vi "Akustische Füllstandsanzeige.vi"() -> ()   [LabVIEW 2018]
uses:
  <vilib>/measure/maspectr.llb/FFT Power Spectrum and PSD for 1 Chan.vi
  <vilib>/measure/NI_MAPro.lvlib
panel:
  out "?":dbl
  out "FFT-Leistung":cluster{"f0":dbl, "df":dbl, "magnitude":dbl[]}(graph)
  in  "Auswahl Gefäß":u16(ring)
  out "?":dbl(slide) scale=0.0..200.0
  in  "?":bool
  # "Füllstand in ml"
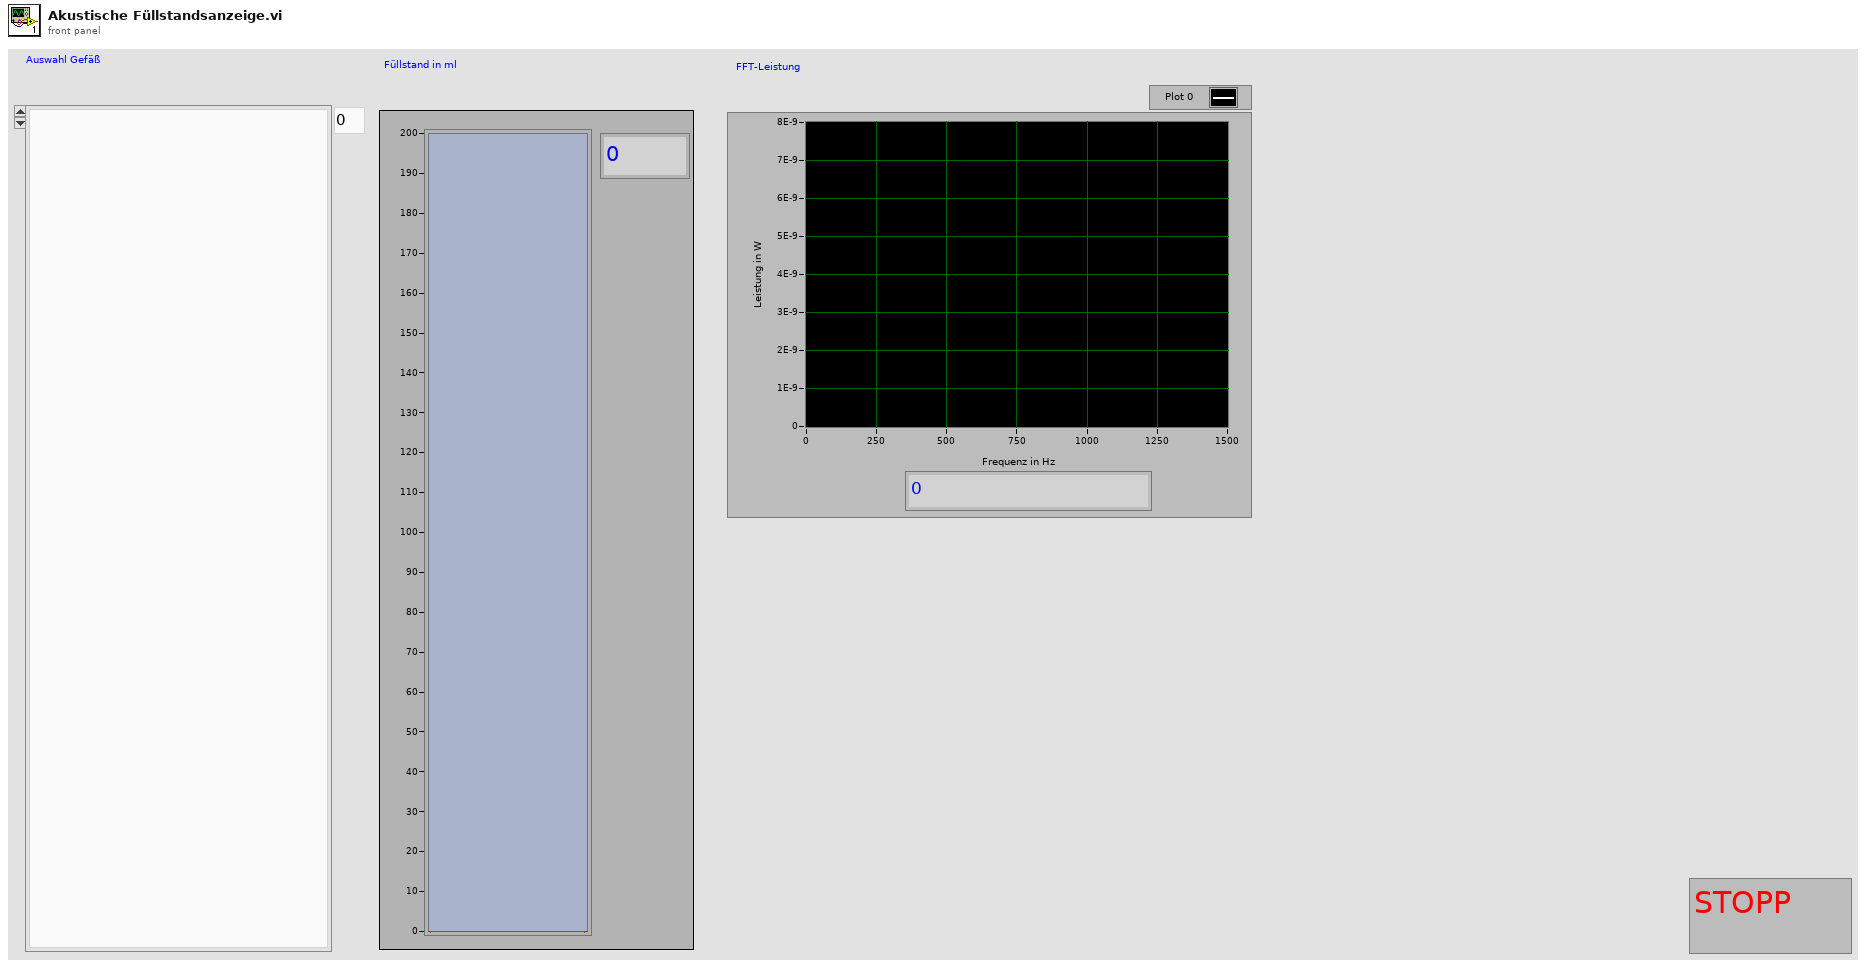
[diagram p1: front panel]
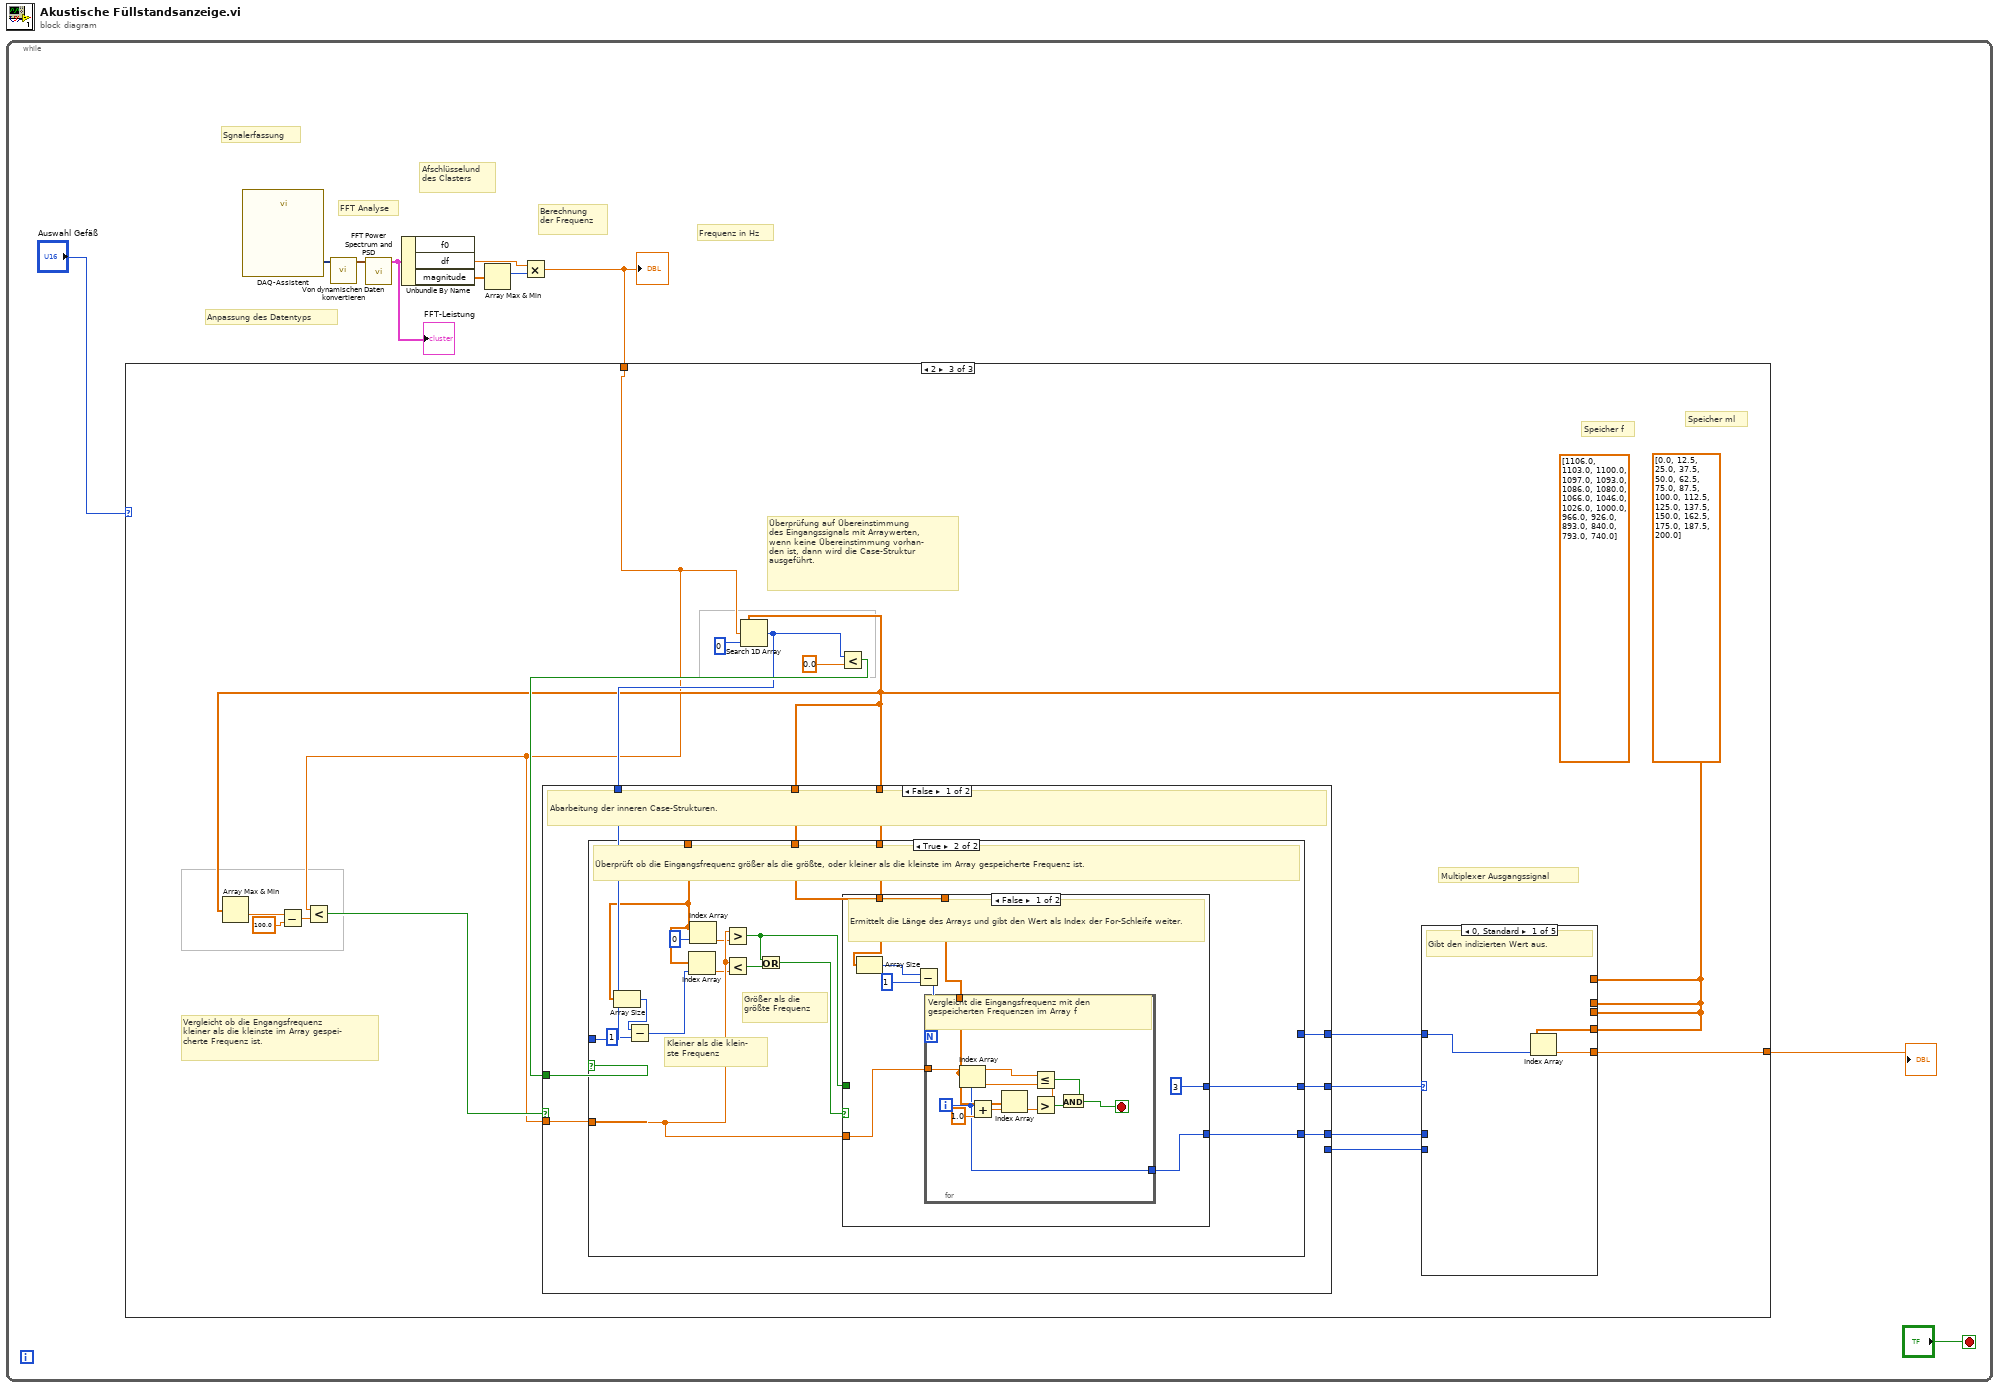
[diagram p0: block diagram]
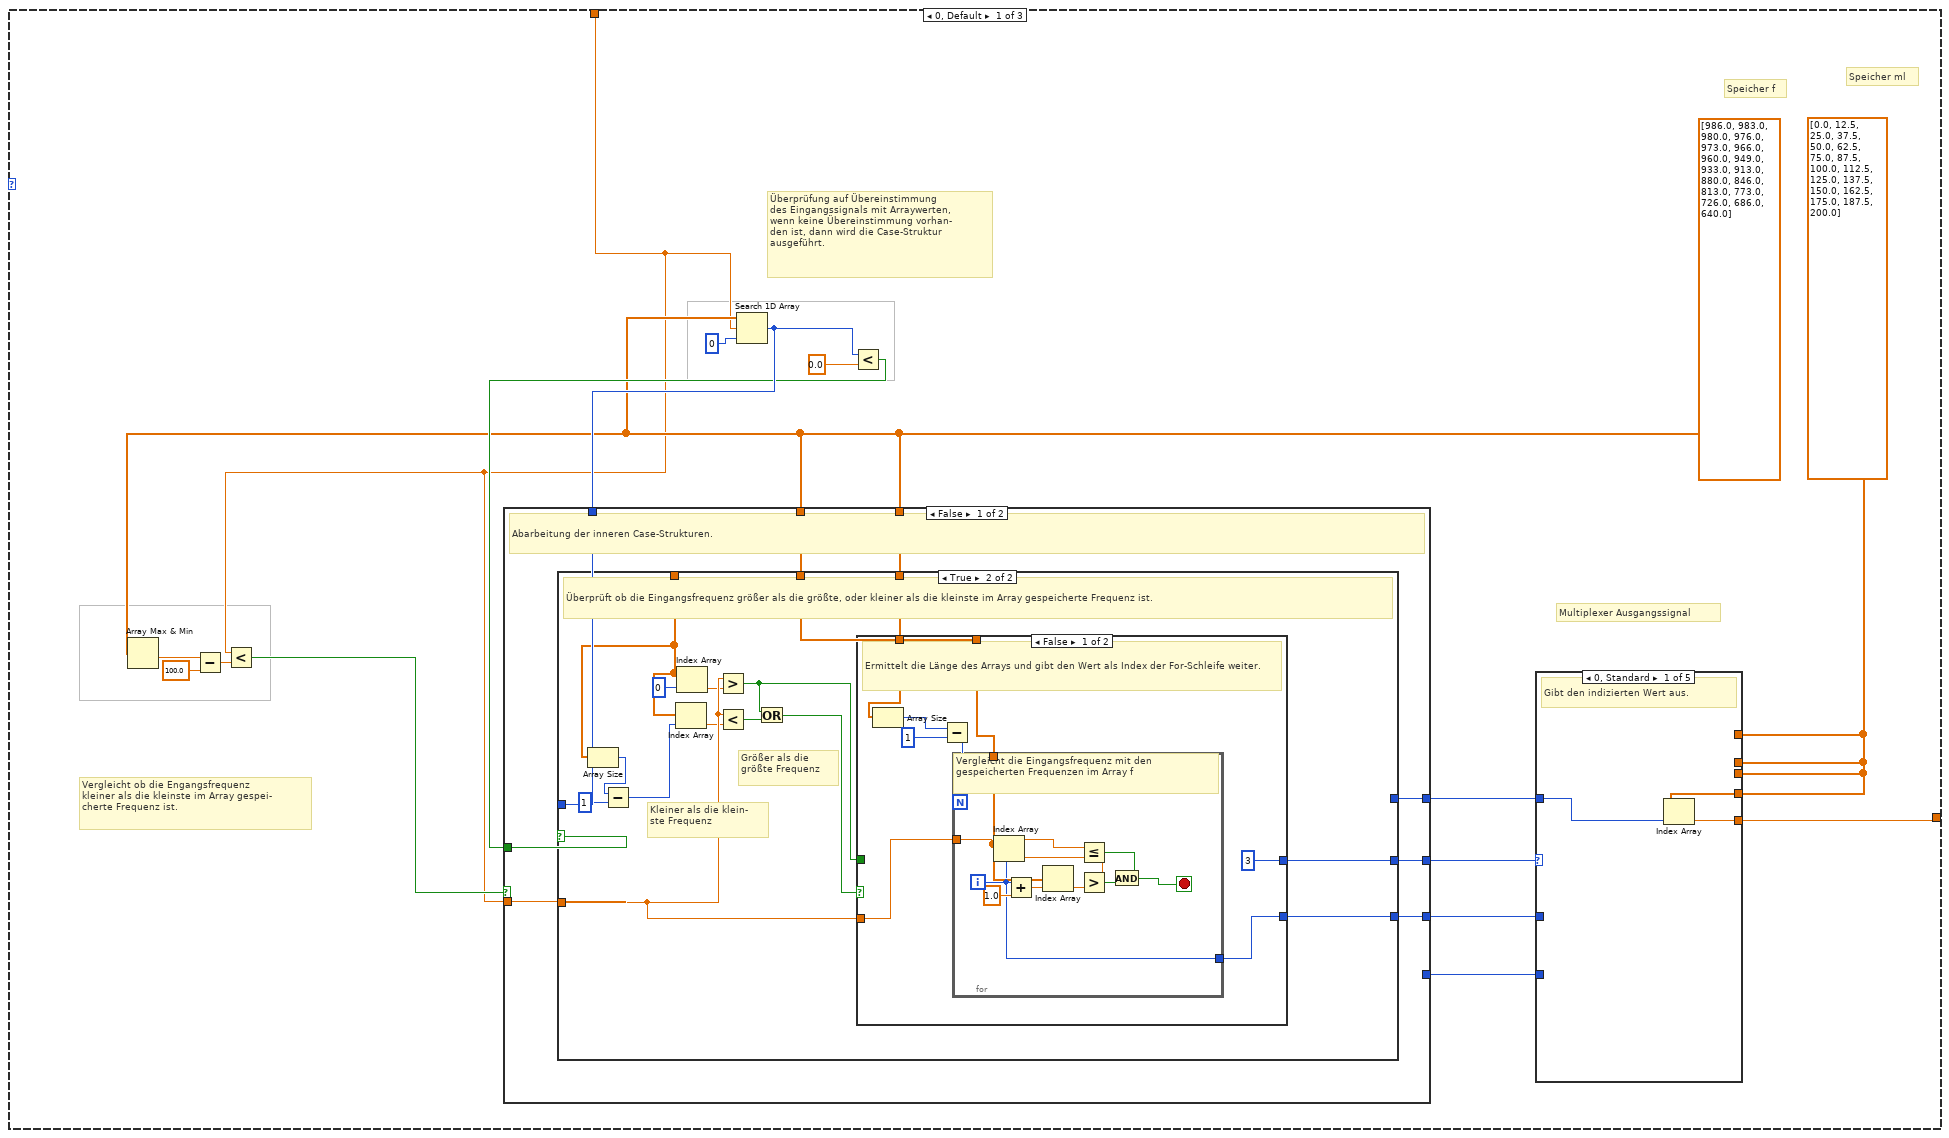
[diagram p2: hidden frame]
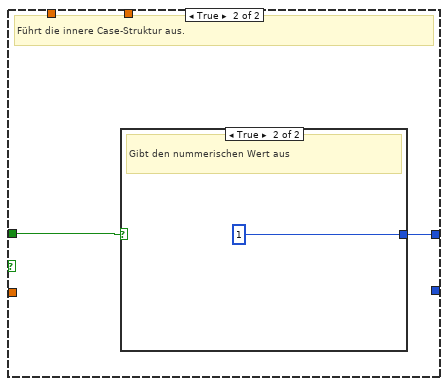
[diagram p4: hidden frame]
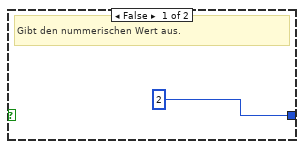
[diagram p5: hidden frame]
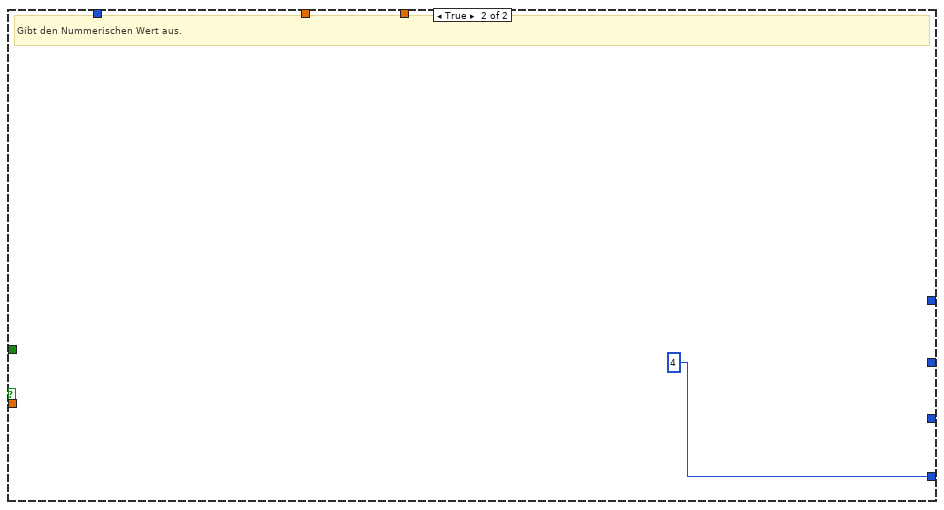
[diagram p6: hidden frame]
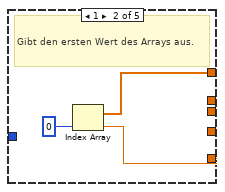
[diagram p7: hidden frame]
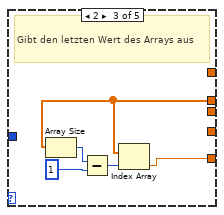
[diagram p8: hidden frame]
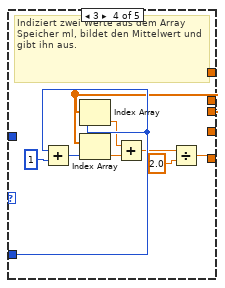
[diagram p9: hidden frame]
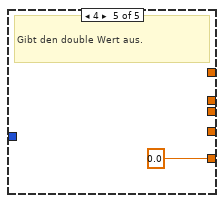
[diagram p10: hidden frame]
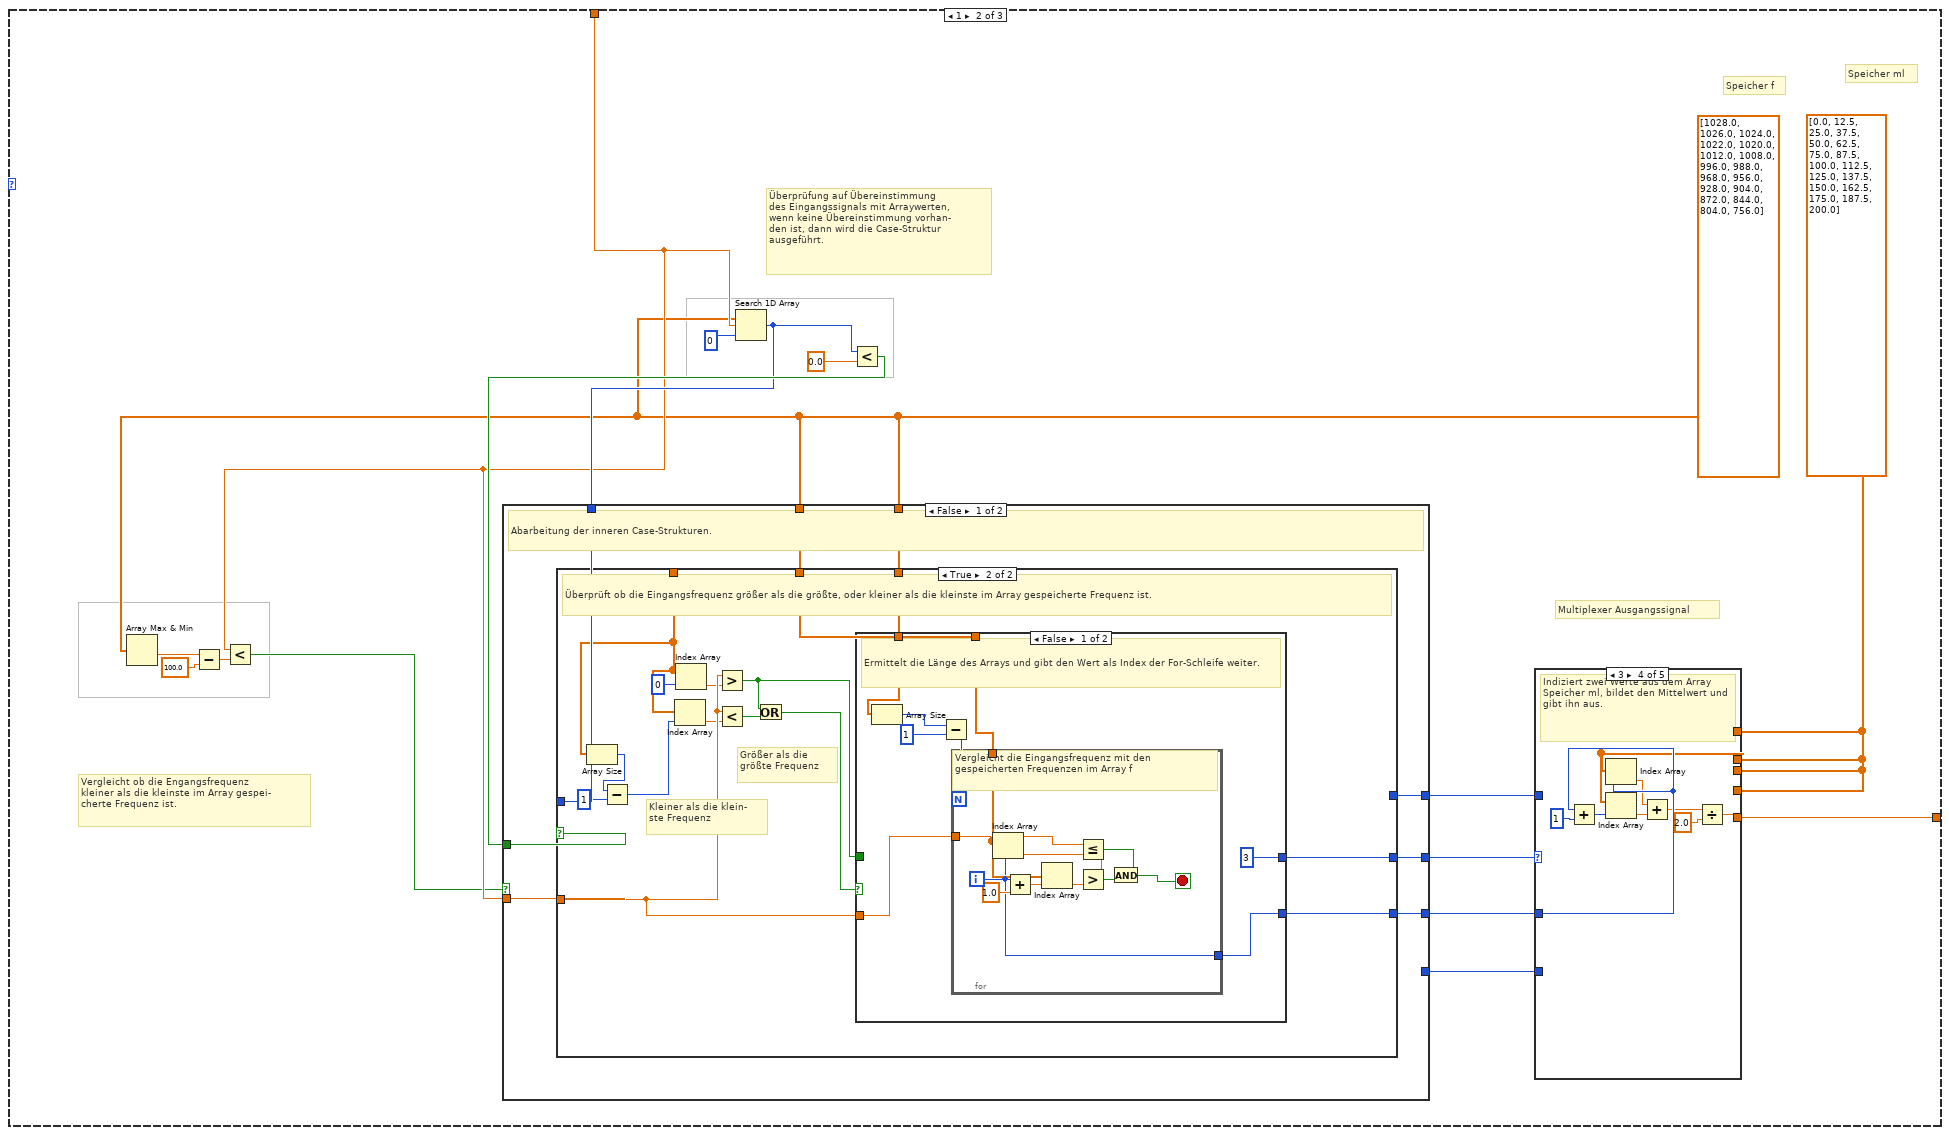
[diagram p11: hidden frame]
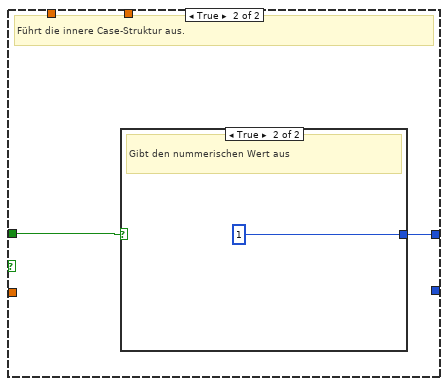
[diagram p13: hidden frame]
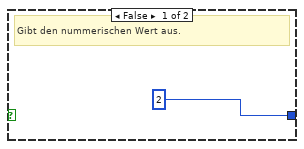
[diagram p14: hidden frame]
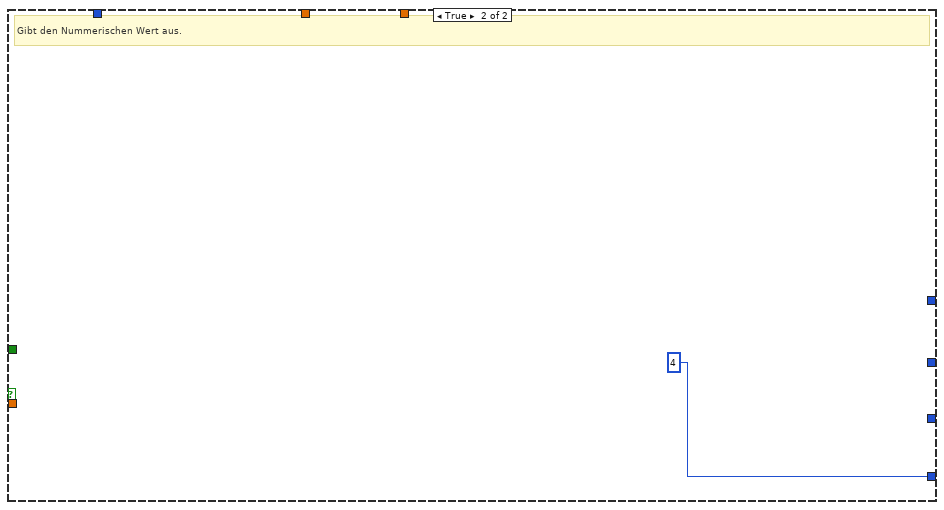
[diagram p15: hidden frame]
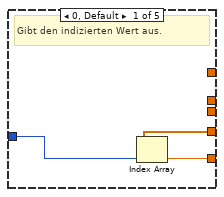
[diagram p16: hidden frame]
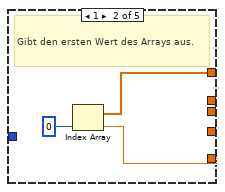
[diagram p17: hidden frame]
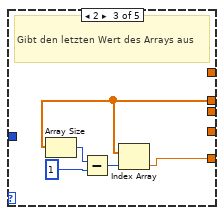
[diagram p18: hidden frame]
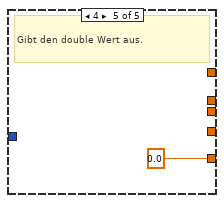
[diagram p19: hidden frame]
diagram:
  n1 = while {
    stop <- "?" stop-if-true
    # "Frequenz in Hz"
    # "Afschlüsselund\ndes Clasters"
    # "Berechnung\nder Frequenz"
    # "FFT Analyse"
    # "Anpassung des Datentyps"
    # "Sgnalerfassung"
    n2 = call "DAQ-Assistent"() -> ("data"=w5:dynamicdata)  [unwired: 16 in, 3 out]
    n3 = call "Von dynamischen Daten konvertieren"("Dynamic Data Type"=w5) -> ("Waveform"=w9:waveform(dbl))  [unwired: 3 in]
    n4 = call-poly <vilib>:"FFT Power Spectrum and PSD.vi"("time signal"=w9) -> ("Power Spectrum / PSD"=w1:cluster{"f0":dbl, "df":dbl, "magnitude":dbl[]})  [unwired: 7 in, 3 out]
    "FFT-Leistung" <- w1
    n5 = Unbundle By Name(w1) -> ("df"=w7:dbl, "magnitude"=w8:dbl[])  [unwired: 1 out]
    n6 = Array Max & Min(array=w8) -> (max index (indices)=w6:i32)  [unwired: 3 out]
    n7 = Multiply(x=w7, y=w6) -> (x*y=w4:dbl)
    "?" <- w4
    n8 = case shown="2" "Auswahl Gefäß" {
      tunnel: w4 -> [w12 w103 w180]
      tunnel: [w11 w96 w179] -> w3
      frame 0, Default {
        w14 = dbl[] [0.0, 12.5, 25.0, 37.5, 50.0, 62.5, 75.0, 87.5, 100.0, 112.5, 125.0, 137.5, 150.0, 162.5, 175.0, 187.5, 200.0]
        w16 = dbl[] [986.0, 983.0, 980.0, 976.0, 973.0, 966.0, 960.0, 949.0, 933.0, 913.0, 880.0, 846.0, 813.0, 773.0, 726.0, 686.0, 640.0]
        # "Überprüfung auf Übereinstimmung\ndes Eingangssignals mit Arraywerten, \nwenn keine Übereinstimmung vorhan-\nden ist, dann wird die Case-Struktur\nausgeführt."
        # "Vergleicht ob die Engangsfrequenz \nkleiner als die kleinste im Array gespei-\ncherte Frequenz ist."
        # "Multiplexer Ausgangssignal"
        # "Speicher ml"
        # "Speicher f"
        n9 = Array Max & Min(array=w16) -> (min value=w22:dbl)  [unwired: 3 out]
        n10 = Subtract(x=w22, y=100.0) -> (x-y=w23:dbl)
        n11 = Less?(x=w12, y=w23) -> (x < y?=w24:bool)
        n12 = Search 1D Array(1D array=w16, element=w12, start index (0)=0 ("Startindex (0)")) -> (index of element=w19:i32)
        n13 = Less?(x=w19, y=0.0) -> (x < y?=w18:bool)
        n14 = case shown="False" w24 {
          tunnel: w18 -> [w34 _]
          tunnel: w19 -> [w33 _]
          tunnel: w12 -> [w32 _]
          tunnel: w16 -> [w31 _]
          tunnel: [w30 _] -> w20
          tunnel: [w29 _] -> w26
          tunnel: [w28 _] -> w21
          tunnel: [_ 4] -> w25
          tunnel: w16 -> [w27 _]
          frame False {
            # "Abarbeitung der inneren Case-Strukturen."
            n15 = case shown="True" w34 {
              tunnel: [w35 _] -> w30
              tunnel: w33 -> [w35 _]
              tunnel: w32 -> [_ w47]
              tunnel: w31 -> [_ w50]
              tunnel: w31 -> [_ w39]
              tunnel: [_ w42] -> w29
              tunnel: [_ w41] -> w28
              tunnel: w27 -> [_ w40]
              frame False {
                # "Schleift den nummerischen Wert durch."
              }
              frame True {
                # "Kleiner als die klein-\nste Frequenz"
                # "Größer als die \ngrößte Frequenz"
                # "Überprüft ob die Eingangsfrequenz größer als die größte, oder kleiner als die kleinste im Array gespeicherte Frequenz ist."
                n16 = Array Size(array=w39) -> (size(s)=w38:i32)
                n17 = Subtract(x=w38, y=1) -> (x-y=w36:i32)
                n18 = Index Array(array=w39, index=w36) -> (element=w45:dbl)
                n19 = Index Array(array=w39, index=0 ("Index")) -> (element=w46:dbl)
                n20 = Greater?(x=w47, y=w46) -> (0:w43:bool)
                n21 = Less?(x=w47, y=w45) -> (x < y?=w49:bool)
                n22 = Or(x=w43, y=w49) -> (x .or. y?=w48:bool)
                n23 = case shown="False" w48 {
                  tunnel: w47 -> [w58 _]
                  tunnel: w50 -> [w57 _]
                  tunnel: w43 -> [_ w70]
                  tunnel: [3 w69] -> w42
                  tunnel: [w55 _] -> w41
                  tunnel: w40 -> [w54 _]
                  frame False {
                    # "Ermittelt die Länge des Arrays und gibt den Wert als Index der For-Schleife weiter."
                    n24 = Array Size(array=w54) -> (size(s)=w53:i32)
                    n25 = Subtract(x=w53, y=1) -> (x-y=w51:i32)
                    n26 = for {
                      N: w51 -> [_]
                      tunnel: w58 -> [w64]
                      tunnel: w57 -> [w65]
                      tunnel: [w59] -> w55
                      i -> [w59]
                      stop <- w60 stop-if-true
                      # "Vergleicht die Eingangsfrequenz mit den gespeicherten Frequenzen im Array f"
                      n27 = Index Array(array=w65, index=w59) -> (element=w66:dbl)
                      n28 = Add(x=w59, y=1.0) -> (x+y=w67:dbl)
                      n29 = Index Array(array=w65, index=w67) -> (element=w63:dbl)
                      n30 = Less Or Equal?(x=w64, y=w66) -> (x <= y?=w61:bool)
                      n31 = Greater?(x=w64, y=w63) -> (0:w62:bool)
                      n32 = And(x=w61, y=w62) -> (x .and. y?=w60:bool)
                    }
                  }
                  frame True {
                    # "Führt die innere Case-Struktur aus."
                    n33 = case shown="True" w70 {
                      tunnel: [2 1] -> w69
                      frame False {
                        # "Gibt den nummerischen Wert aus."
                      }
                      frame True {
                        # "Gibt den nummerischen Wert aus"
                      }
                    }
                  }
                }
              }
            }
          }
          frame True {
            # "Gibt den Nummerischen Wert aus."
          }
        }
        n34 = case shown="0, Standard" w26 {
          tunnel: w14 -> [w76 _ _ _ _]
          tunnel: w20 -> [w75 _ _ _ _]
          tunnel: w14 -> [_ w79 _ _ _]
          tunnel: [w74 w77 w84 w85 0.0] -> w11
          tunnel: w14 -> [_ _ w83 _ _]
          tunnel: w21 -> [_ _ _ w93 _]
          tunnel: w14 -> [_ _ _ w90 _]
          tunnel: w25 -> [_ _ _ _ _]
          frame 0, Default {
            # "Gibt den indizierten Wert aus."
            n35 = Index Array(array=w76, index=w75) -> (element=w74:dbl)
          }
          frame 1 {
            # "Gibt den ersten Wert des Arrays aus."
            n36 = Index Array(array=w79, index=0 ("Index")) -> (element=w77:dbl)
          }
          frame 2 {
            # "Gibt den letzten Wert des Arrays aus"
            n37 = Array Size(array=w83) -> (size(s)=w82:i32)
            n38 = Subtract(x=w82, y=1) -> (x-y=w80:i32)
            n39 = Index Array(array=w83, index=w80) -> (element=w84:dbl)
          }
          frame 3 {
            # "Indiziert zwei Werte aus dem Array Speicher ml, bildet den Mittelwert und gibt ihn aus."
            n40 = Add(x=w93, y=1) -> (x+y=w91:i32)
            n41 = Index Array(array=w90, index=w93) -> (element=w89:dbl)
            n42 = Index Array(array=w90, index=w91) -> (element=w88:dbl)
            n43 = Add(x=w89, y=w88) -> (x+y=w87:dbl)
            n44 = Divide(x=w87, y=2.0) -> (x/y=w85:dbl)
          }
          frame 4 {
            # "Gibt den double Wert aus."
          }
        }
      }
      frame 1 {
        w104 = dbl[] [0.0, 12.5, 25.0, 37.5, 50.0, 62.5, 75.0, 87.5, 100.0, 112.5, 125.0, 137.5, 150.0, 162.5, 175.0, 187.5, 200.0]
        w97 = dbl[] [1028.0, 1026.0, 1024.0, 1022.0, 1020.0, 1012.0, 1008.0, 996.0, 988.0, 968.0, 956.0, 928.0, 904.0, 872.0, 844.0, 804.0, 756.0]
        # "Überprüfung auf Übereinstimmung\ndes Eingangssignals mit Arraywerten, \nwenn keine Übereinstimmung vorhan-\nden ist, dann wird die Case-Struktur\nausgeführt."
        # "Vergleicht ob die Engangsfrequenz \nkleiner als die kleinste im Array gespei-\ncherte Frequenz ist."
        # "Multiplexer Ausgangssignal"
        # "Speicher ml"
        # "Speicher f"
        n45 = Array Max & Min(array=w97) -> (min value=w102:dbl)  [unwired: 3 out]
        n46 = Subtract(x=w102, y=100.0) -> (x-y=w100:dbl)
        n47 = Less?(x=w103, y=w100) -> (x < y?=w99:bool)
        n48 = Search 1D Array(1D array=w97, element=w103, start index (0)=0 ("Startindex (0)")) -> (index of element=w107:i32)
        n49 = Less?(x=w107, y=0.0) -> (x < y?=w108:bool)
        n50 = case shown="False" w99 {
          tunnel: w108 -> [w118 _]
          tunnel: w107 -> [w117 _]
          tunnel: w103 -> [w116 _]
          tunnel: w97 -> [w115 _]
          tunnel: [w114 _] -> w106
          tunnel: [w113 _] -> w95
          tunnel: [w112 _] -> w105
          tunnel: [_ 4] -> w98
          tunnel: w97 -> [w111 _]
          frame False {
            # "Abarbeitung der inneren Case-Strukturen."
            n51 = case shown="True" w118 {
              tunnel: [w119 _] -> w114
              tunnel: w117 -> [w119 _]
              tunnel: w116 -> [_ w131]
              tunnel: w115 -> [_ w134]
              tunnel: w115 -> [_ w123]
              tunnel: [_ w126] -> w113
              tunnel: [_ w125] -> w112
              tunnel: w111 -> [_ w124]
              frame False {
                # "Schleift den nummerischen Wert durch."
              }
              frame True {
                # "Kleiner als die klein-\nste Frequenz"
                # "Größer als die \ngrößte Frequenz"
                # "Überprüft ob die Eingangsfrequenz größer als die größte, oder kleiner als die kleinste im Array gespeicherte Frequenz ist."
                n52 = Array Size(array=w123) -> (size(s)=w122:i32)
                n53 = Subtract(x=w122, y=1) -> (x-y=w120:i32)
                n54 = Index Array(array=w123, index=w120) -> (element=w129:dbl)
                n55 = Index Array(array=w123, index=0 ("Index")) -> (element=w130:dbl)
                n56 = Greater?(x=w131, y=w130) -> (0:w127:bool)
                n57 = Less?(x=w131, y=w129) -> (x < y?=w133:bool)
                n58 = Or(x=w127, y=w133) -> (x .or. y?=w132:bool)
                n59 = case shown="False" w132 {
                  tunnel: w131 -> [w142 _]
                  tunnel: w134 -> [w141 _]
                  tunnel: w127 -> [_ w154]
                  tunnel: [3 w153] -> w126
                  tunnel: [w139 _] -> w125
                  tunnel: w124 -> [w138 _]
                  frame False {
                    # "Ermittelt die Länge des Arrays und gibt den Wert als Index der For-Schleife weiter."
                    n60 = Array Size(array=w138) -> (size(s)=w137:i32)
                    n61 = Subtract(x=w137, y=1) -> (x-y=w135:i32)
                    n62 = for {
                      N: w135 -> [_]
                      tunnel: w142 -> [w148]
                      tunnel: w141 -> [w149]
                      tunnel: [w143] -> w139
                      i -> [w143]
                      stop <- w144 stop-if-true
                      # "Vergleicht die Eingangsfrequenz mit den gespeicherten Frequenzen im Array f"
                      n63 = Index Array(array=w149, index=w143) -> (element=w150:dbl)
                      n64 = Add(x=w143, y=1.0) -> (x+y=w151:dbl)
                      n65 = Index Array(array=w149, index=w151) -> (element=w147:dbl)
                      n66 = Less Or Equal?(x=w148, y=w150) -> (x <= y?=w145:bool)
                      n67 = Greater?(x=w148, y=w147) -> (0:w146:bool)
                      n68 = And(x=w145, y=w146) -> (x .and. y?=w144:bool)
                    }
                  }
                  frame True {
                    # "Führt die innere Case-Struktur aus."
                    n69 = case shown="True" w154 {
                      tunnel: [2 1] -> w153
                      frame False {
                        # "Gibt den nummerischen Wert aus."
                      }
                      frame True {
                        # "Gibt den nummerischen Wert aus"
                      }
                    }
                  }
                }
              }
            }
          }
          frame True {
            # "Gibt den Nummerischen Wert aus."
          }
        }
        n70 = case shown="3" w95 {
          tunnel: w104 -> [w160 _ _ _ _]
          tunnel: w106 -> [w159 _ _ _ _]
          tunnel: w104 -> [_ w163 _ _ _]
          tunnel: [w158 w161 w168 w169 0.0] -> w96
          tunnel: w104 -> [_ _ w167 _ _]
          tunnel: w105 -> [_ _ _ w177 _]
          tunnel: w104 -> [_ _ _ w174 _]
          tunnel: w98 -> [_ _ _ _ _]
          frame 0, Default {
            # "Gibt den indizierten Wert aus."
            n71 = Index Array(array=w160, index=w159) -> (element=w158:dbl)
          }
          frame 1 {
            # "Gibt den ersten Wert des Arrays aus."
            n72 = Index Array(array=w163, index=0 ("Index")) -> (element=w161:dbl)
          }
          frame 2 {
            # "Gibt den letzten Wert des Arrays aus"
            n73 = Array Size(array=w167) -> (size(s)=w166:i32)
            n74 = Subtract(x=w166, y=1) -> (x-y=w164:i32)
            n75 = Index Array(array=w167, index=w164) -> (element=w168:dbl)
          }
          frame 3 {
            # "Indiziert zwei Werte aus dem Array Speicher ml, bildet den Mittelwert und gibt ihn aus."
            n76 = Add(x=w177, y=1) -> (x+y=w175:i32)
            n77 = Index Array(array=w174, index=w177) -> (element=w173:dbl)
            n78 = Index Array(array=w174, index=w175) -> (element=w172:dbl)
            n79 = Add(x=w173, y=w172) -> (x+y=w171:dbl)
            n80 = Divide(x=w171, y=2.0) -> (x/y=w169:dbl)
          }
          frame 4 {
            # "Gibt den double Wert aus."
          }
        }
      }
      frame 2 {
        w188 = dbl[] [0.0, 12.5, 25.0, 37.5, 50.0, 62.5, 75.0, 87.5, 100.0, 112.5, 125.0, 137.5, 150.0, 162.5, 175.0, 187.5, 200.0]
        w182 = dbl[] [1106.0, 1103.0, 1100.0, 1097.0, 1093.0, 1086.0, 1080.0, 1066.0, 1046.0, 1026.0, 1000.0, 966.0, 926.0, 893.0, 840.0, 793.0, 740.0]
        # "Überprüfung auf Übereinstimmung\ndes Eingangssignals mit Arraywerten, \nwenn keine Übereinstimmung vorhan-\nden ist, dann wird die Case-Struktur\nausgeführt."
        # "Vergleicht ob die Engangsfrequenz \nkleiner als die kleinste im Array gespei-\ncherte Frequenz ist."
        # "Multiplexer Ausgangssignal"
        # "Speicher ml"
        # "Speicher f"
        n81 = Array Max & Min(array=w182) -> (min value=w187:dbl)  [unwired: 3 out]
        n82 = Subtract(x=w187, y=100.0) -> (x-y=w185:dbl)
        n83 = Less?(x=w180, y=w185) -> (x < y?=w184:bool)
        n84 = Search 1D Array(1D array=w182, element=w180, start index (0)=0 ("Startindex (0)")) -> (index of element=w191:i32)
        n85 = Less?(x=w191, y=0.0) -> (x < y?=w192:bool)
        n86 = case shown="False" w184 {
          tunnel: w192 -> [w202 _]
          tunnel: w191 -> [w201 _]
          tunnel: w180 -> [w200 _]
          tunnel: w182 -> [w199 _]
          tunnel: [w198 _] -> w190
          tunnel: [w197 _] -> w181
          tunnel: [w196 _] -> w189
          tunnel: [_ 4] -> w183
          tunnel: w182 -> [w195 _]
          frame False {
            # "Abarbeitung der inneren Case-Strukturen."
            n87 = case shown="True" w202 {
              tunnel: [w203 _] -> w198
              tunnel: w201 -> [w203 _]
              tunnel: w200 -> [_ w215]
              tunnel: w199 -> [_ w218]
              tunnel: w199 -> [_ w207]
              tunnel: [_ w210] -> w197
              tunnel: [_ w209] -> w196
              tunnel: w195 -> [_ w208]
              frame False {
                # "Schleift den nummerischen Wert durch."
              }
              frame True {
                # "Kleiner als die klein-\nste Frequenz"
                # "Größer als die \ngrößte Frequenz"
                # "Überprüft ob die Eingangsfrequenz größer als die größte, oder kleiner als die kleinste im Array gespeicherte Frequenz ist."
                n88 = Array Size(array=w207) -> (size(s)=w206:i32)
                n89 = Subtract(x=w206, y=1) -> (x-y=w204:i32)
                n90 = Index Array(array=w207, index=w204) -> (element=w213:dbl)
                n91 = Index Array(array=w207, index=0 ("Index")) -> (element=w214:dbl)
                n92 = Greater?(x=w215, y=w214) -> (0:w211:bool)
                n93 = Less?(x=w215, y=w213) -> (x < y?=w217:bool)
                n94 = Or(x=w211, y=w217) -> (x .or. y?=w216:bool)
                n95 = case shown="False" w216 {
                  tunnel: w215 -> [w226 _]
                  tunnel: w218 -> [w225 _]
                  tunnel: w211 -> [_ w238]
                  tunnel: [3 w237] -> w210
                  tunnel: [w223 _] -> w209
                  tunnel: w208 -> [w222 _]
                  frame False {
                    # "Ermittelt die Länge des Arrays und gibt den Wert als Index der For-Schleife weiter."
                    n96 = Array Size(array=w222) -> (size(s)=w221:i32)
                    n97 = Subtract(x=w221, y=1) -> (x-y=w219:i32)
                    n98 = for {
                      N: w219 -> [_]
                      tunnel: w226 -> [w232]
                      tunnel: w225 -> [w233]
                      tunnel: [w227] -> w223
                      i -> [w227]
                      stop <- w228 stop-if-true
                      # "Vergleicht die Eingangsfrequenz mit den gespeicherten Frequenzen im Array f"
                      n99 = Index Array(array=w233, index=w227) -> (element=w234:dbl)
                      n100 = Add(x=w227, y=1.0) -> (x+y=w235:dbl)
                      n101 = Index Array(array=w233, index=w235) -> (element=w231:dbl)
                      n102 = Less Or Equal?(x=w232, y=w234) -> (x <= y?=w229:bool)
                      n103 = Greater?(x=w232, y=w231) -> (0:w230:bool)
                      n104 = And(x=w229, y=w230) -> (x .and. y?=w228:bool)
                    }
                  }
                  frame True {
                    # "Führt die innere Case-Struktur aus."
                    n105 = case shown="True" w238 {
                      tunnel: [2 1] -> w237
                      frame False {
                        # "Gibt den nummerischen Wert aus."
                      }
                      frame True {
                        # "Gibt den nummerischen Wert aus"
                      }
                    }
                  }
                }
              }
            }
          }
          frame True {
            # "Gibt den Nummerischen Wert aus."
          }
        }
        n106 = case shown="0, Standard" w181 {
          tunnel: w188 -> [w244 _ _ _ _]
          tunnel: w190 -> [w243 _ _ _ _]
          tunnel: w188 -> [_ w247 _ _ _]
          tunnel: [w242 w245 w252 w253 0.0] -> w179
          tunnel: w188 -> [_ _ w251 _ _]
          tunnel: w189 -> [_ _ _ w261 _]
          tunnel: w188 -> [_ _ _ w258 _]
          tunnel: w183 -> [_ _ _ _ _]
          frame 0, Default {
            # "Gibt den indizierten Wert aus."
            n107 = Index Array(array=w244, index=w243) -> (element=w242:dbl)
          }
          frame 1 {
            # "Gibt den ersten Wert des Arrays aus."
            n108 = Index Array(array=w247, index=0 ("Index")) -> (element=w245:dbl)
          }
          frame 2 {
            # "Gibt den letzten Wert des Arrays aus"
            n109 = Array Size(array=w251) -> (size(s)=w250:i32)
            n110 = Subtract(x=w250, y=1) -> (x-y=w248:i32)
            n111 = Index Array(array=w251, index=w248) -> (element=w252:dbl)
          }
          frame 3 {
            # "Indiziert zwei Werte aus dem Array Speicher ml, bildet den Mittelwert und gibt ihn aus."
            n112 = Add(x=w261, y=1) -> (x+y=w259:i32)
            n113 = Index Array(array=w258, index=w261) -> (element=w257:dbl)
            n114 = Index Array(array=w258, index=w259) -> (element=w256:dbl)
            n115 = Add(x=w257, y=w256) -> (x+y=w255:dbl)
            n116 = Divide(x=w255, y=2.0) -> (x/y=w253:dbl)
          }
          frame 4 {
            # "Gibt den double Wert aus."
          }
        }
      }
    }
    "?" <- w3
  }
